vi "Error Size.vi"(11 "error size":T1=enum."512") -> (2 "power of 2":i16, 3 "size":u64 format="%d bytes")   [LabVIEW 2017, in "DSF Core.lvlib" / "Error Pointer.lvclass"]
uses:
  Error Pointer.lvclass
  Error Sizes.ctl
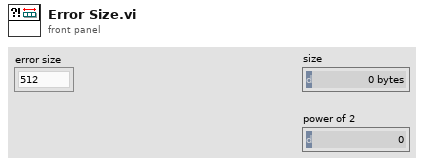
[diagram p1: front panel]
types:
  T1 = typedef "DSF Core.lvlib/Error Pointer.lvclass/Error Sizes.ctl" = enum8{"256", "512", "1024"}
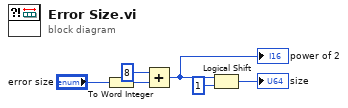
[diagram p0: block diagram]
diagram:
  n1 = To Word Integer(number="error size") -> (16bit integer=w4:i16)
  n2 = Add(x=i16 8 ("y"), y=w4) -> (x+y=w1:i16)
  "power of 2" <- w1
  n3 = Logical Shift(y=w1, x=u64 1) -> (x << y=→"size":u64)
